vi "ResetFirmware.vi"(3 "error in":errorcluster, 4 "listing in":string, 5 "connection ID in":refnum<k5>) -> (0 "error out":errorcluster, 1 "listing out":string, 2 "connection ID":refnum<k5>)   [LabVIEW 2009]
panel:
  # "This LabVIEW item is deprecated.\n\nIt is believed to be unused and will be removed in a future version of SRV."
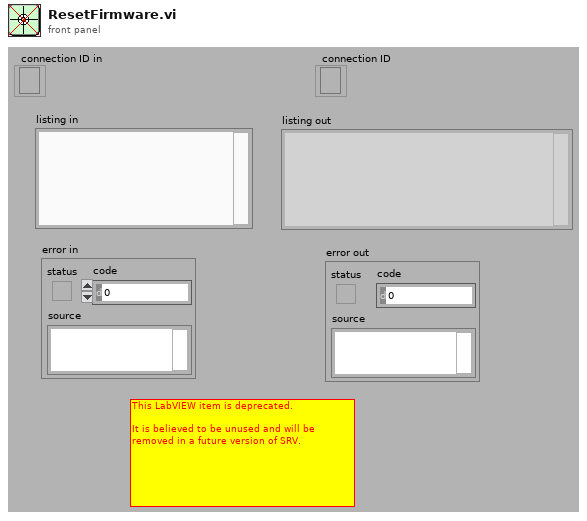
[diagram p1: front panel]
types:
  T1 = cluster{"bytes to read":i32, "msec pause":u32, "msec timeout":i32}
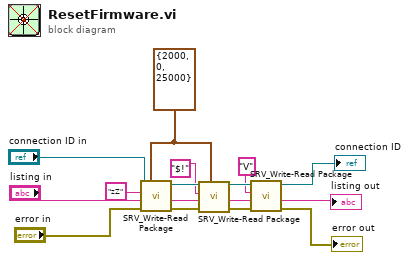
[diagram p0: block diagram]
diagram:
  w3 = T1 {"bytes to read"=2000, "msec pause"=0, "msec timeout"=25000} ("parameters")
  n1 = call "SRV_Write-Read Package.vi"("parameters"=w3, "error in"="error in", "listing in"="listing in", "data in"="zZ", "connection ID in"="connection ID in") -> ("error out"=w11:errorcluster, "listing out"=w10:string, "connection ID"=w13:refnum<k5>)  [unwired: 3 in, 1 out]
  n2 = call "SRV_Write-Read Package.vi"("parameters"=w3, "error in"=w11, "listing in"=w10, "data in"="$!", "connection ID in"=w13) -> ("error out"=w9:errorcluster, "listing out"=w8:string, "connection ID"=w7:refnum<k5>)  [unwired: 3 in, 1 out]
  n3 = call "SRV_Write-Read Package.vi"("error in"=w9, "listing in"=w8, "data in"="V", "connection ID in"=w7) -> ("error out"=→"error out":errorcluster, "listing out"=→"listing out":string, "connection ID"=→"connection ID":refnum<k5>)  [unwired: 4 in, 1 out]
